vi "myRIO_BRig_Host_v0,09.vi"() -> ()   [LabVIEW 2014]
panel:
  out "RunTime_minutes":u16
  out "RunTime_seconds":u16
  out "error out 2":errorcluster caption="error out"
  in  "dataIn_maxTrialsDisplayed":u16 caption="Number of Trials Displayed\n( 0 = all trials )"
  in  "colorIn_timeout":u32(colorbox)=7468543 caption="Choice Timeout"
  in  "colorIn_wrong/cue":u32(colorbox)=16728618 caption="Wrong Choice or\nLicked During Cue"
  in  "colorIn_reward":u32(colorbox)=5898088 caption="Reward"
  in  "colorIn_unknown":u32(colorbox)=16449331 caption="Unknown Trial Status"
  in  "LoadPrevSettings":bool
  out "BlockL_BTPR_cur":u16 caption="BadTrialsPostReward"
  out "BlockL_T2R_cur":u16 caption="Trials2Reward"
  out "BlockL_BTPR_avg":dbl caption="BadTrialsPostReward" format="%#_3g"
  out "BlockL_T2R_avg":dbl caption="Trials2Reward" format="%#_3g"
  out "BlockR_BTPR_cur":u16 caption="BadTrialsPostReward"
  out "BlockR_T2R_cur":u16 caption="Trials2Reward"
  out "BlockR_BTPR_avg":dbl caption="BadTrialsPostReward" format="%#_3g"
  out "BlockR_T2R_avg":dbl caption="Trials2Reward" format="%#_3g"
  out "dataOut_plot":cluster{i32[], i32[]}[](graph)
  out "iBlock":u16
  out "iTrial":u16
  in  "stop":bool
  # "Exp Stats"
  # "Current Block Stats"
  # "Trials 2 Reward\n\nBad Trials\nPost Reward"
  # "Left Spout    Right Spout"
  # "Run Time\n\n   minutes    seconds"
  # "Average Block Stats"
  # "Trials 2 Reward\n\nBad Trials\nPost Reward"
  # "Left Spout    Right Spout"
  # "If you get ERROR 5 related to opening a file, press CONTINUE"
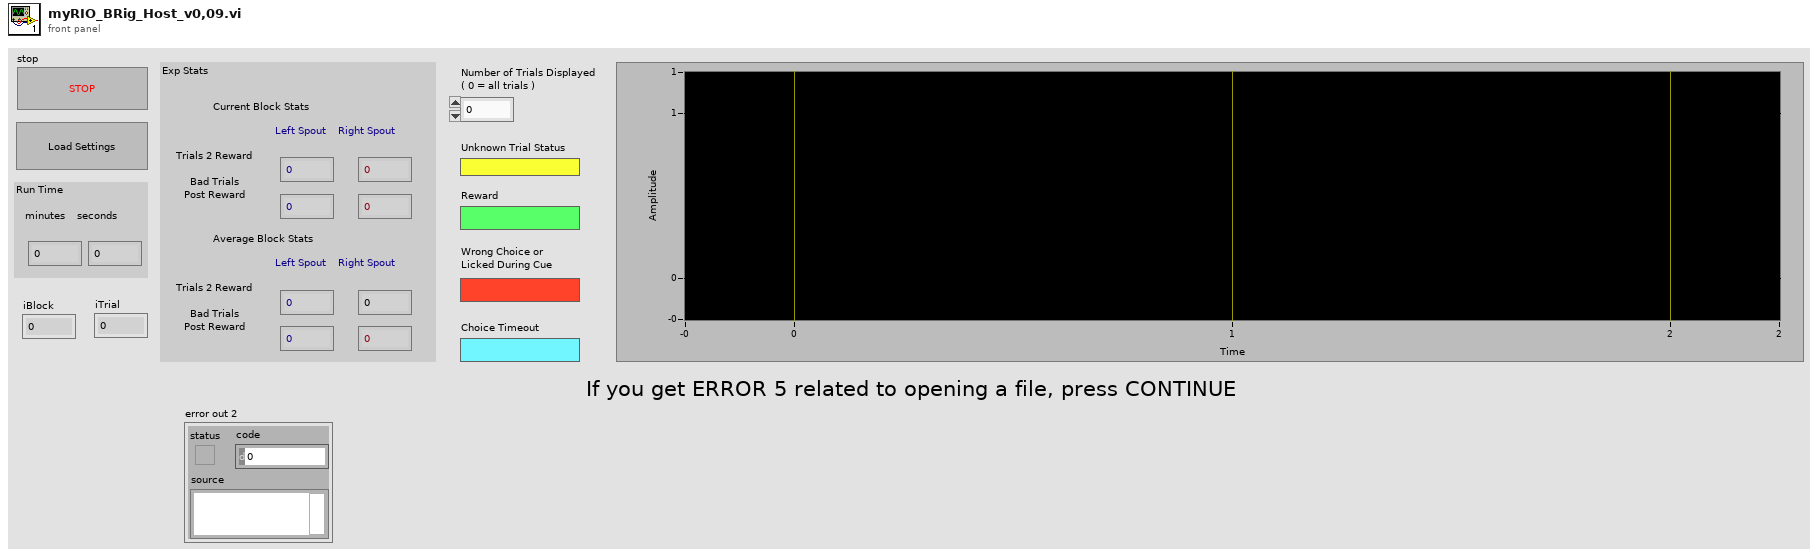
[diagram p1: front panel]
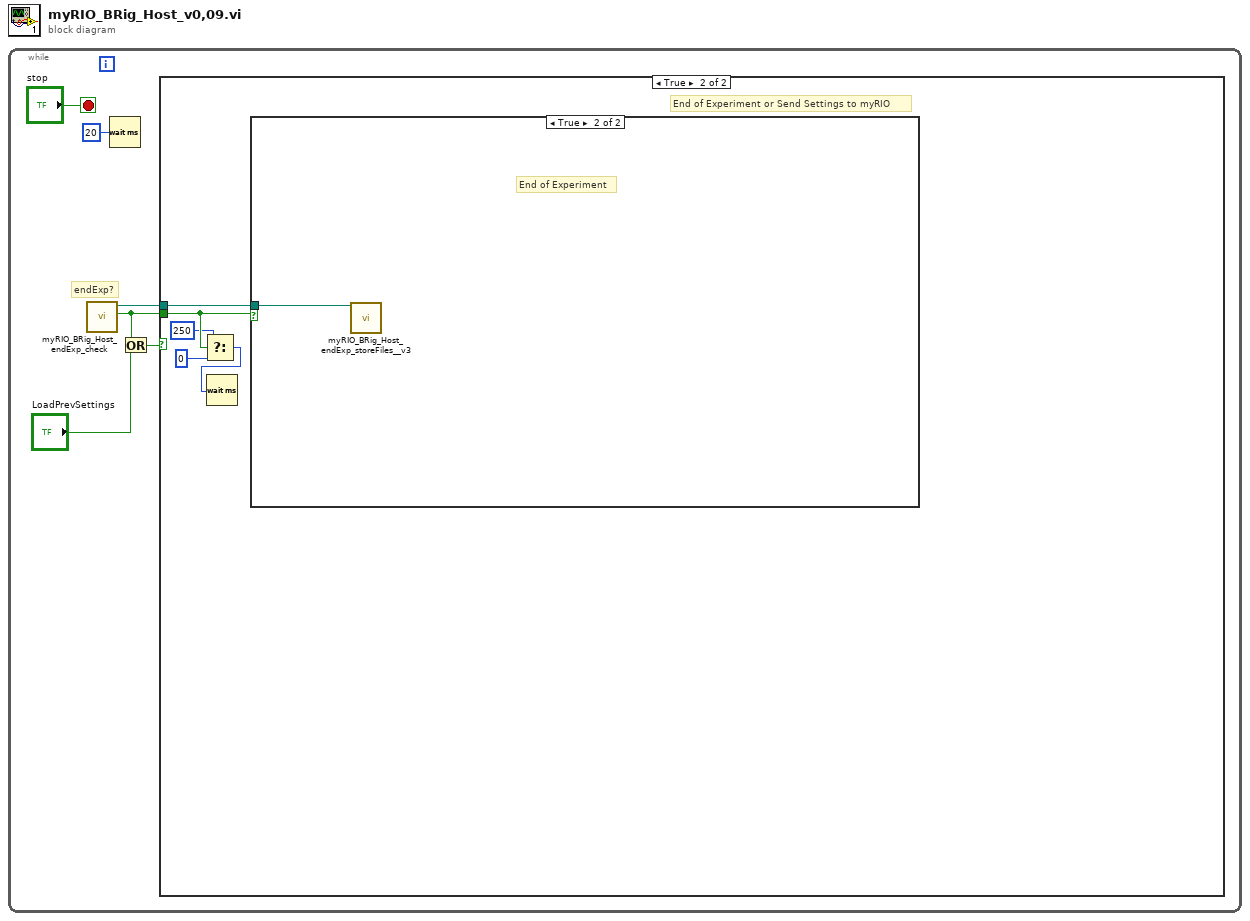
[diagram p0: block diagram]
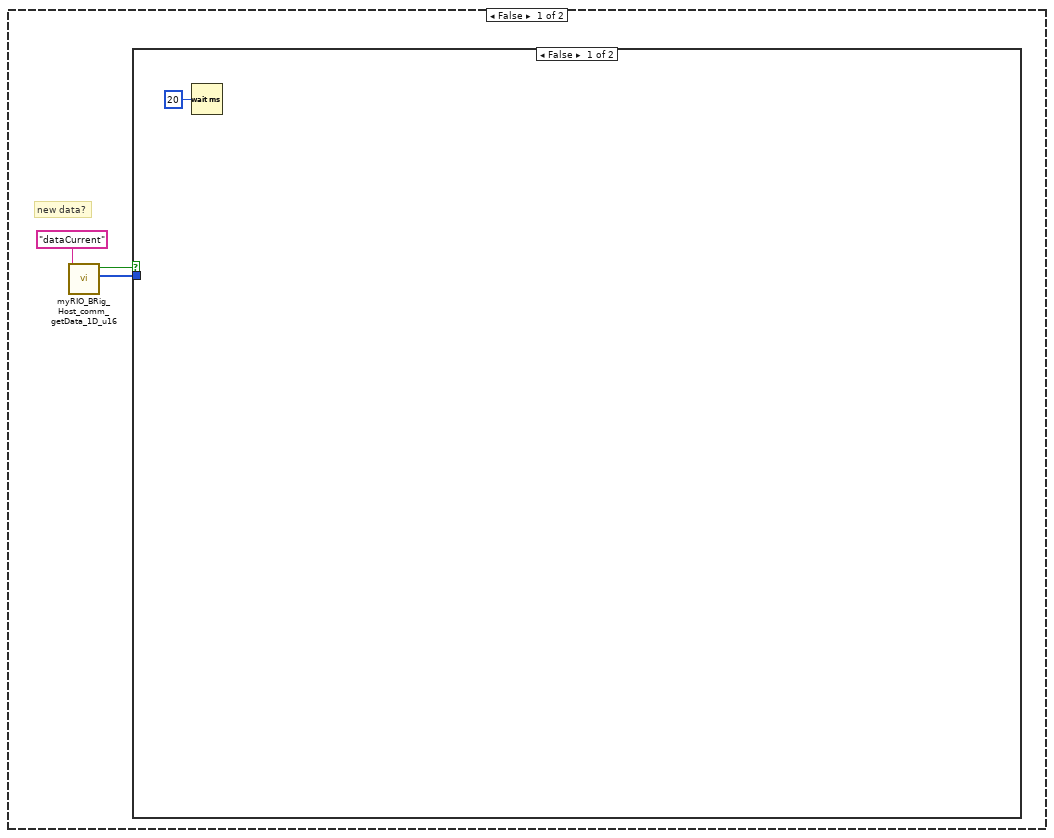
[diagram p2: hidden frame]
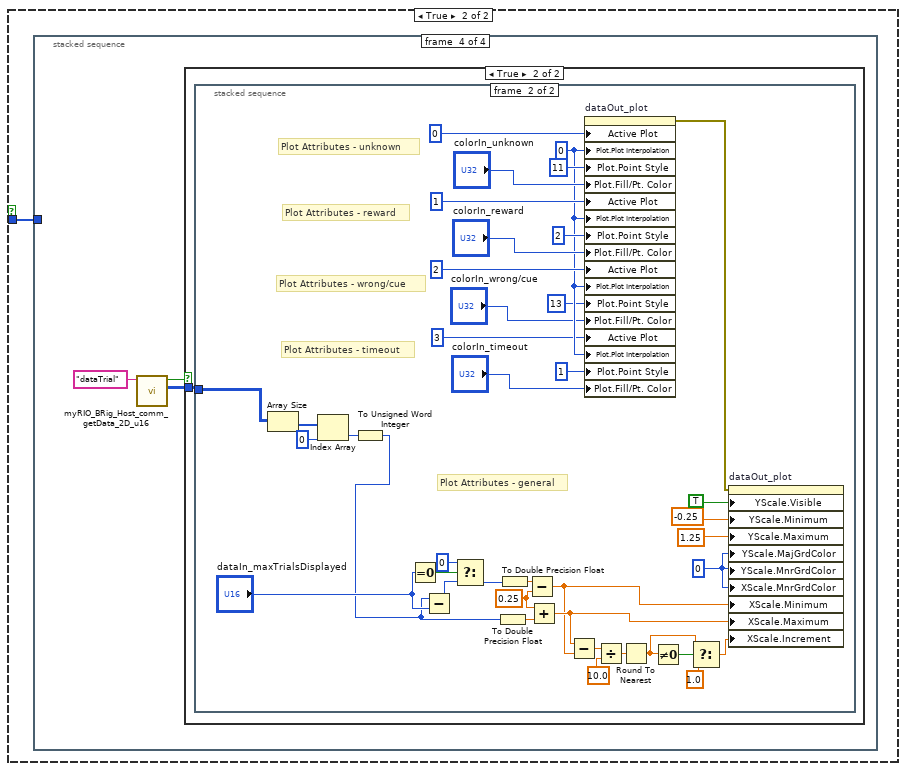
[diagram p3: hidden frame]
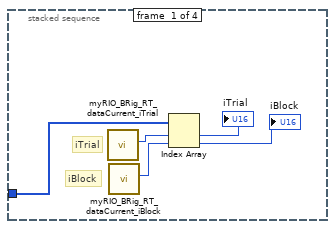
[diagram p4: hidden frame]
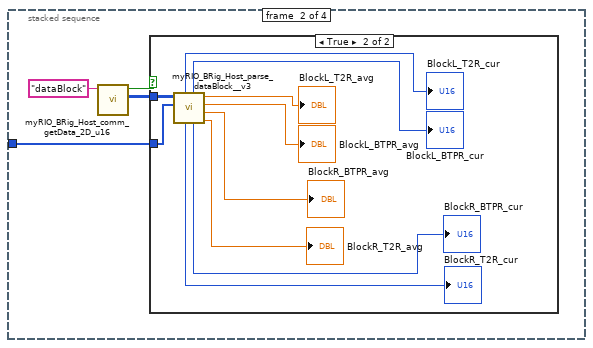
[diagram p5: hidden frame]
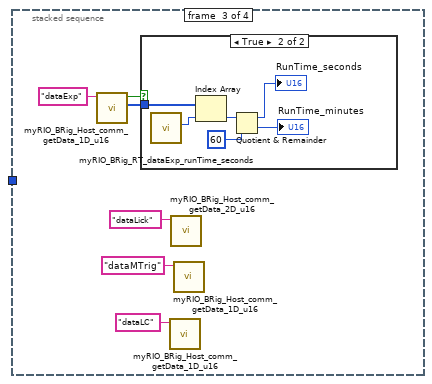
[diagram p7: hidden frame]
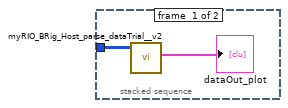
[diagram p10: hidden frame]
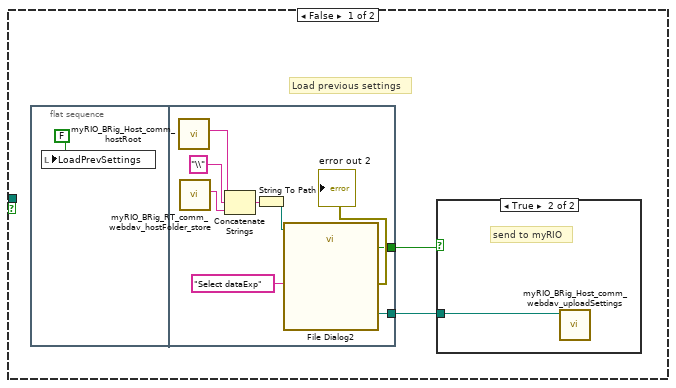
[diagram p11: hidden frame]
diagram:
  n1 = while {
    stop <- "stop" stop-if-true
    # "endExp?"
    n2 = call "myRIO_BRig_Host_endExp_check.vi"() -> ("output_IendExp"=w3:bool, "output_filePath_expExp"=w2:path)  [unwired: 10 in]
    n3 = Wait (ms)(milliseconds to wait=u32 20) -> ()  [unwired: 1 out]
    n4 = Or(x=w3, y="LoadPrevSettings") -> (x .or. y?=w4:bool)
    n5 = case shown="True" w4 {
      tunnel: w3 -> [_ w92]
      tunnel: w2 -> [_ w93]
      frame False {
        # "new data?"
        n6 = call "myRIO_BRig_Host_comm_getData_1D_u16.vi"("input_fileName"="dataCurrent") -> ("output_data_1D"=w7:u16[], "output_I_data"=w8:bool)  [unwired: 9 in]
        n7 = case shown="False" w8 {
          tunnel: w7 -> [_ w11]
          frame False {
            n8 = Wait (ms)(milliseconds to wait=u32 20) -> ()  [unwired: 1 out]
          }
          frame True {
            n9 = stacked-sequence {
              tunnel: w11 -> [w12 w17 _ _]
              frame #0 {
                # "iBlock"
                # "iTrial"
                n10 = call "myRIO_BRig_RT_dataCurrent_iTrial.vi"() -> ("output_iTrial"=w16:i32)  [unwired: 11 in]
                n11 = call "myRIO_BRig_RT_dataCurrent_iBlock.vi"() -> ("output_iBlock"=w15:i32)  [unwired: 11 in]
                n12 = Index Array(array=w12, index #1=w16, index #2=w15) -> (element #1=→"iTrial":u16, element #2=→"iBlock":u16)
              }
              frame #1 {
                n13 = call "myRIO_BRig_Host_comm_getData_2D_u16.vi"("input_fileName"="dataBlock") -> ("output_data_2D"=w18:u16[][], "output_I_data"=w19:bool)  [unwired: 9 in]
                n14 = case shown="True" w19 {
                  tunnel: w18 -> [_ w22]
                  tunnel: w17 -> [_ w21]
                  frame False {
                  }
                  frame True {
                    n15 = call "myRIO_BRig_Host_parse_dataBlock__v3.vi"("input_dataCurrent"=w21, "input_dataBlock"=w22) -> ("BlockR_T2R_avg"=→"BlockR_T2R_avg":dbl, "BlockR_BTPR_avg"=→"BlockR_BTPR_avg":dbl, "BlockL_BTPR_avg"=→"BlockL_BTPR_avg":dbl, "BlockL_T2R_avg"=→"BlockL_T2R_avg":dbl, "BlockR_BTPR_cur"=→"BlockR_BTPR_cur":u16, "BlockL_BTPR_cur"=→"BlockL_BTPR_cur":u16, "BlockR_T2R_cur"=→"BlockR_T2R_cur":u16, "BlockL_T2R_cur"=→"BlockL_T2R_cur":u16)  [unwired: 2 in]
                  }
                }
              }
              frame #2 {
                n16 = call "myRIO_BRig_Host_comm_getData_1D_u16.vi"("input_fileName"="dataExp") -> ("output_data_1D"=w34:u16[], "output_I_data"=w35:bool)  [unwired: 9 in]
                n17 = case shown="True" w35 {
                  tunnel: w34 -> [_ w42]
                  frame False {
                  }
                  frame True {
                    n18 = call "myRIO_BRig_RT_dataExp_runTime_seconds.vi"() -> ("output_RunTime_minutes"=w41:i32)  [unwired: 11 in]
                    n19 = Index Array(array=w42, index=w41) -> (element=w40:u16)
                    n20 = Quotient & Remainder(x=w40, y=u16 60) -> (x-y*floor(x/y)=→"RunTime_seconds":u16, floor(x/y)=→"RunTime_minutes":u16)
                  }
                }
                n21 = call "myRIO_BRig_Host_comm_getData_1D_u16.vi"("input_fileName"="dataLC") -> ()  [unwired: 9 in, 2 out]
                n22 = call "myRIO_BRig_Host_comm_getData_2D_u16.vi"("input_fileName"="dataLick") -> ()  [unwired: 9 in, 2 out]
                n23 = call "myRIO_BRig_Host_comm_getData_1D_u16.vi"("input_fileName"="dataMTrig") -> ()  [unwired: 9 in, 2 out]
              }
              frame #3 {
                n24 = call "myRIO_BRig_Host_comm_getData_2D_u16.vi"("input_fileName"="dataTrial") -> ("output_data_2D"=w44:u16[][], "output_I_data"=w43:bool)  [unwired: 9 in]
                n25 = case shown="True" w43 {
                  tunnel: w44 -> [_ w46]
                  frame False {
                  }
                  frame True {
                    n26 = stacked-sequence {
                      tunnel: w46 -> [w47 w53]
                      frame #0 {
                        n27 = call "myRIO_BRig_Host_parse_dataTrial__v2.vi"("arrayIn_dataTrial"=w47) -> ("appended array"=→"dataOut_plot":cluster{i32[], i32[]}[])  [unwired: 10 in]
                      }
                      frame #1 {
                        w68 = 0.25 ("y")
                        w72 = u32 0 ("Y Scale.Grid Colors:Major Color")
                        w81 = u8 0 ("Plot.Plot Interpolation")
                        # "Plot Attributes - general"
                        # "Plot Attributes - timeout"
                        # "Plot Attributes - wrong/cue"
                        # "Plot Attributes - reward"
                        # "Plot Attributes - unknown"
                        n28 = Array Size(array=w53) -> (size(s)=w55:i32[])
                        n29 = Index Array(array=w55, index=0) -> (element=w51:i32)
                        n30 = To Unsigned Word Integer(number=w51) -> (unsigned 16bit integer=w50:u16)
                        n31 = Equal To 0?(x="dataIn_maxTrialsDisplayed") -> (x = 0?=w71:bool)
                        n32 = Subtract(x=w50, y="dataIn_maxTrialsDisplayed") -> (x-y=w70:u16)
                        n33 = Select(t=u16 0, s=w71, f=w70) -> (s? t:f=w65:u16)
                        n34 = To Double Precision Float(number=w50) -> (double precision float=w67:dbl)
                        n35 = To Double Precision Float(number=w65) -> (double precision float=w66:dbl)
                        n36 = Subtract(x=w66, y=w68) -> (x-y=w57:dbl)
                        n37 = Add(x=w68, y=w67) -> (x+y=w58:dbl)
                        n38 = Subtract(x=w58, y=w57) -> (x-y=w64:dbl)
                        n39 = property on="dataOut_plot" class="XYGraph (strict)"("Active Plot"=u32 0, "Plot.Plot Interpolation"=w81, "Plot.Point Style"=u8 11, "Plot.Fill/Pt. Color"="colorIn_unknown", "Active Plot"=u32 1, "Plot.Plot Interpolation"=w81, "Plot.Point Style"=u8 2, "Plot.Fill/Pt. Color"="colorIn_reward", "Active Plot"=u32 2, "Plot.Plot Interpolation"=w81, "Plot.Point Style"=u8 13, "Plot.Fill/Pt. Color"="colorIn_wrong/cue", "Active Plot"=u32 3, "Plot.Plot Interpolation"=w81, "Plot.Point Style"=u8 1, "Plot.Fill/Pt. Color"="colorIn_timeout") -> (error out=w56:errorcluster)  [unwired: 2 in, 1 out]
                        n40 = Divide(x=w64, y=10.0) -> (x/y=w62:dbl)
                        n41 = Round To Nearest(number=w62) -> (nearest integer value=w60:dbl)
                        n42 = Not Equal To 0?(x=w60) -> (x != 0?=w61:bool)
                        n43 = Select(t=w60, s=w61, f=1.0) -> (s? t:f=w59:dbl)
                        n44 = property on="dataOut_plot" class="XYGraph (strict)"(error in=w56, "YScale.Visible"=TRUE ("Y Scale.Visible"), "YScale.Minimum"=-0.25 ("Y Scale.Range:Minimum"), "YScale.Maximum"=1.25 ("Y Scale.Range:Maximum"), "YScale.MajGrdColor"=w72, "YScale.MnrGrdColor"=w72, "XScale.MnrGrdColor"=w72, "XScale.Minimum"=w57, "XScale.Maximum"=w58, "XScale.Increment"=w59) -> ()  [unwired: 1 in, 2 out]
                      }
                    }
                  }
                }
              }
            }
          }
        }
      }
      frame True {
        # "End of Experiment or Send Settings to myRIO"
        n45 = Select(t=u32 250 ("milliseconds to wait"), s=w92, f=u32 0 ("milliseconds to wait")) -> (s? t:f=w90:u32)
        n46 = Wait (ms)(milliseconds to wait=w90) -> ()  [unwired: 1 out]
        n47 = case shown="True" w92 {
          tunnel: w93 -> [_ w107]
          frame False {
            # "Load previous settings"
            n48 = flat-sequence {
              tunnel: [w99] -> w94
              tunnel: [w98] -> w95
              frame #0 {
                n49 = local write "LoadPrevSettings"(FALSE ("LoadPrevSettings")) -> ()
              }
              frame #1 {
                n50 = call "myRIO_BRig_Host_comm_hostRoot.vi"() -> ("output_hostRoot"=w101:string)  [unwired: 11 in]
                n51 = call "myRIO_BRig_RT_comm_webdav_hostFolder_store.vi"() -> ("output_HostFolder"=w103:string)  [unwired: 11 in]
                n52 = Concatenate Strings(w101, "\\" ("string"), w103) -> (w105:string)
                n53 = String To Path(string=w105) -> (path=w104:path)
                n54 = call "File Dialog2"("start path"=w104, "prompt"="Select dataExp") -> ("selected path"=w99:path, "exists"=w98:bool, "error out"=→"error out 2":errorcluster)  [unwired: 10 in, 1 out]
              }
            }
            n55 = case shown="True" w95 {
              tunnel: w94 -> [_ w96]
              frame False {
                # "invalid file\nor\ncancelled"
              }
              frame True {
                # "send to myRIO"
                n56 = call "myRIO_BRig_Host_comm_webdav_uploadSettings.vi"("input_filePath"=w96) -> ()  [unwired: 11 in]
              }
            }
          }
          frame True {
            # "End of Experiment"
            n57 = call "myRIO_BRig_Host_endExp_storeFiles__v3.vi"("input_filePath"=w107) -> ()  [unwired: 15 in]
          }
        }
      }
    }
  }
